vi "TIFF-Stack-Subtract.vi"() -> ()   [LabVIEW 2011]
uses:
  Library/tiff/TiffModules/AddTiffPage_U16_text_res.vi
panel:
  in  "Subtract":path
  out "Page":i32
  in  "Output file":u16(ring)=257 items=["Big-Endian"=0, "Native"=1, "Little-Endian"=2, "BigTiff-Big-Endian"=256, "Bigtiff,Native"=257, "Biftiff,Littleendian"=258]
  in  "inputfile-Stack":path
  in  "Stop at offset:":u64=429496729500
  out "AfterDIRoffset":u32 format="%09d"
  out "Out":u16[][](graph)
  out "In":u16[][](graph)
  # "Name-offset.tif"
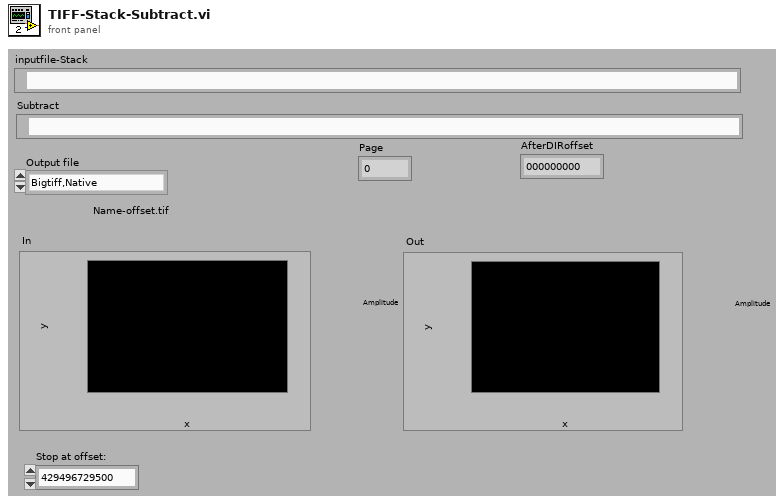
[diagram p1: front panel]
types:
  T1 = cluster{"Tiff refnum":refnum<file>, "BigTiff,Endian":u16}
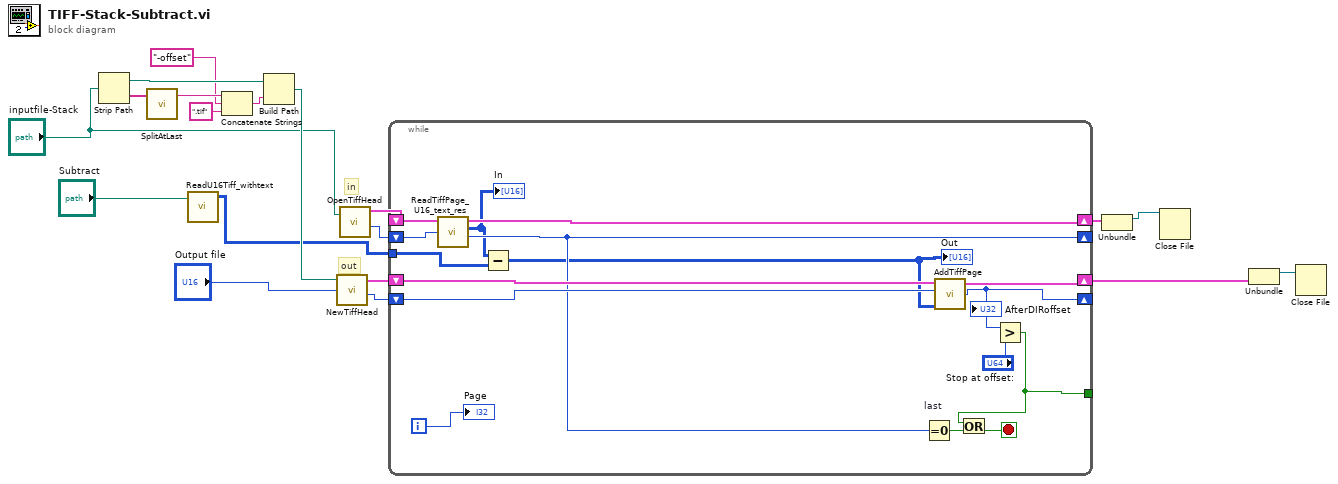
[diagram p0: block diagram]
diagram:
  # "out"
  # "in"
  n1 = Strip Path(path="inputfile-Stack") -> (stripped path=w11:path, name=w12:string)
  n2 = call "SplitAtLast.vi"("In-String"=w12) -> ("Front (default)"=w13:string)  [unwired: 1 in, 1 out]
  n3 = call "ReadU16Tiff_withtext.vi"("file path"="Subtract") -> ("I16 pixmap"=w1:u16[][])  [unwired: 1 in, 2 out]
  n4 = Concatenate Strings(w13, "-offset" ("string"), ".tif" ("string")) -> (w19:string)
  n5 = Build Path(base path=w11, name or relative path=w19) -> (appended path=w18:path)
  n6 = call "NewTiffHead.vi"("file path"=w18, "BigTiff,Endian"="Output file") -> ("TIFF file"=w17:T1, "Place for first IFD (8,eof-position)"=w16:u64)  [unwired: 2 in, 1 out]
  n7 = call "OpenTiffHead.vi"("file path"="inputfile-Stack") -> ("TIFF file"=w8:T1, "first Diroffset"=w7:u64)  [unwired: 2 in, 1 out]
  n8 = while {
    shift-right: [w29] -> w6
    shift-left: w8 -> [w31]
    shift-right: [w34] -> w15
    shift-left: w17 -> [w35]
    shift-right: [w24] -> _
    shift-left: w7 -> [w30]
    shift-right: [w25] -> _
    shift-left: w16 -> [w33]
    tunnel: [w26] -> _
    tunnel: w1 -> [w21]
    i -> [w23]
    stop <- w27 stop-if-true
    n9 = call "ReadTiffPage_U16_text_res.vi"("TIFF file"=w31, "IFDoffset"=w30) -> ("TIFF file out"=w29:T1, "16-bit pixmap"=w22:u16[][], "Next offset"=w24:i64)  [unwired: 3 in, 3 out]
    "In" <- w22
    n10 = Subtract(x=w22, y=w21) -> (x-y=w20:u16[][])
    "Out" <- w20
    n11 = Equal To 0? "last"(x=w24) -> (x = 0?=w32:bool)
    n12 = call-poly "AddTiffPage.vi"("TIFF file"=w35, "After last DIROffset"=w33, "16-bit pixmap x, y"=w20) -> ("TIFF file"=w34:T1, "AfterDIRoffset"=w25:u64)  [unwired: 2 in, 1 out]
    "AfterDIRoffset" <- w25
    n13 = Greater?(x=w25, y="Stop at offset:") -> (0:w26:bool)
    n14 = Or(x=w26, y=w32) -> (x .or. y?=w27:bool)
    "Page" <- w23
  }
  n15 = Unbundle(w6) -> ("Tiff refnum"=w5:refnum<file>)  [unwired: 1 out]
  n16 = Close File(refnum=w5) -> ()  [unwired: 1 in, 2 out]
  n17 = Unbundle(w15) -> ("Tiff refnum"=w14:refnum<file>)  [unwired: 1 out]
  n18 = Close File(refnum=w14) -> ()  [unwired: 1 in, 2 out]
